vi "Qualify Library Icon Core.vi"(0 "VI Reference":refnum<vi>, 11 "error in":errorcluster) -> (3 "Class?":bool, 4 "Good Library Icon":bool, 6 "Maximum Number of Rows":i32, 8 "Library Path":path, 10 "Number of Rows in Icon":i32, 14 "Icon Image":picture, 15 "error out":errorcluster)   [LabVIEW 2020, in "Text-Based VI Icon.lvlib"]
uses:
  Text-Based VI Icon.lvlib
panel:
  out "Left and Right Good (for Debugging)":bool
  out "Top and Bottom Good (for Debugging)":bool
  out "Good Frame Color (for Debugging)":bool
  out "Supported Size or Shape (for Debugging)":bool
  out "Last True Mask + 1 (for Debugging)":i32
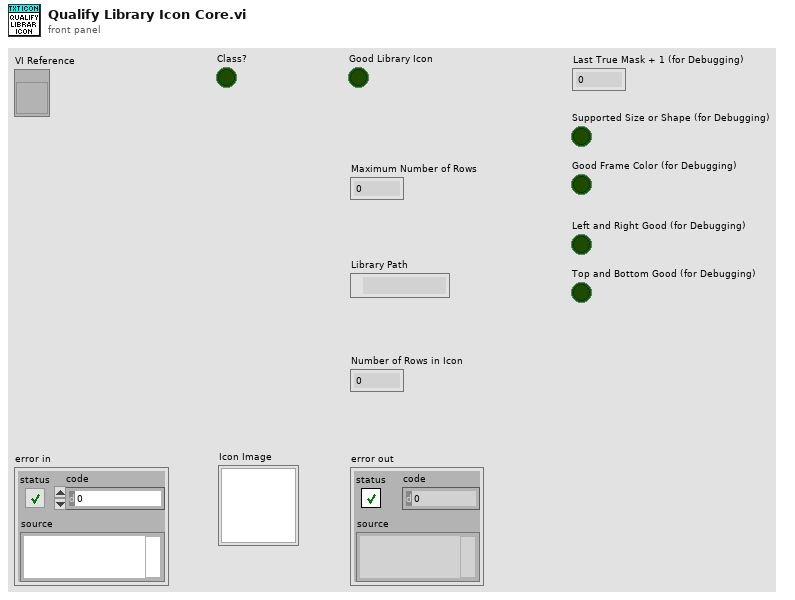
[diagram p1: front panel]
types:
  T1 = typedef "imagedata.ctl" = cluster{"image type":i32, "image depth":i32, "image":u8[], "mask":u8[], "colors":u32[], "Rectangle":cluster{"left":i16, "top":i16, "right":i16, "bottom":i16}}
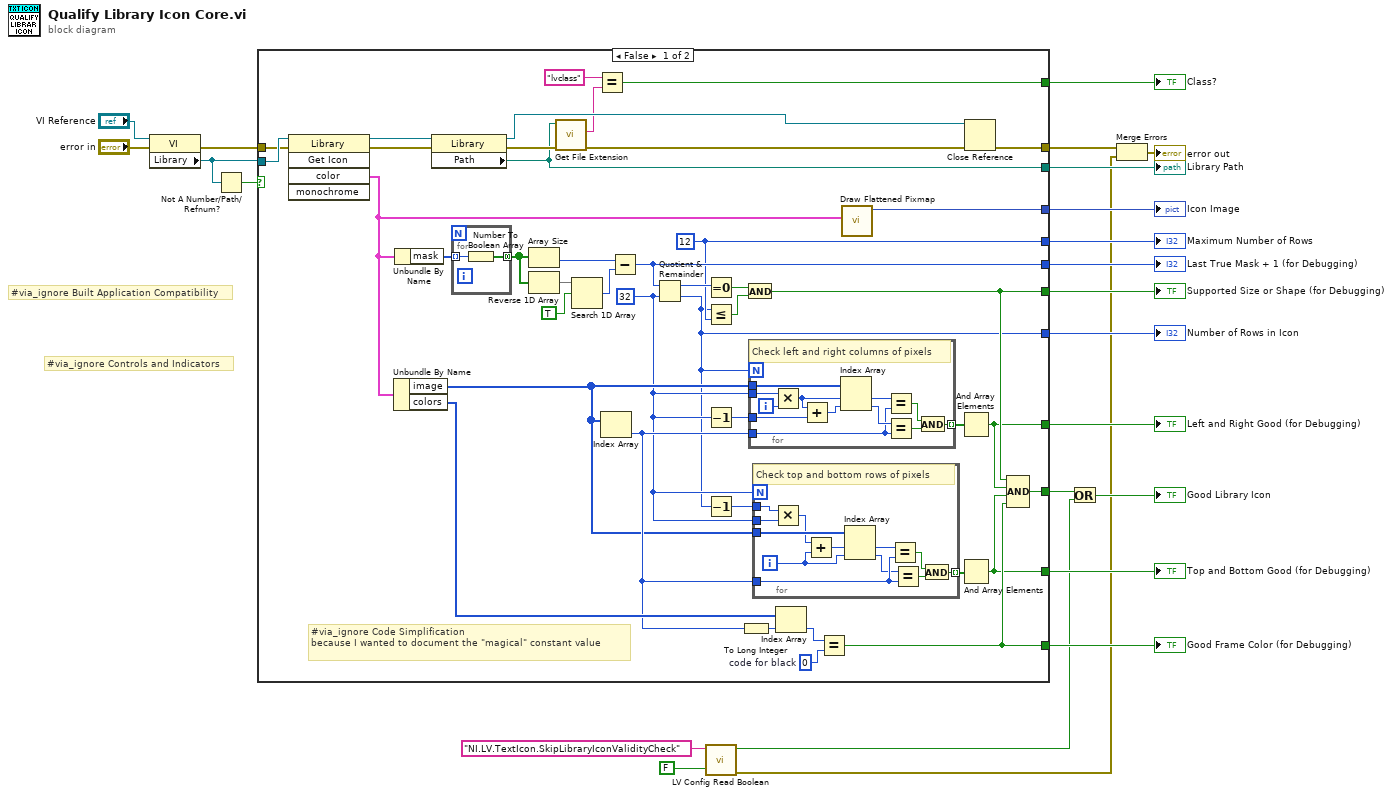
[diagram p0: block diagram]
diagram:
  # "#via_ignore Built Application Compatibility"
  # "#via_ignore Controls and Indicators"
  n1 = property class="VI"(reference="VI Reference", error in="error in") -> (error out=w21:errorcluster, "Library"=w22:refnum<vi>)  [unwired: 1 out]
  n2 = Not A Number/Path/Refnum?(number/path/refnum=w22) -> (NaN/Path/Refnum?=w23:bool)
  n3 = case shown="False" w23 {
    tunnel: w22 -> [w65 _]
    tunnel: w21 -> [w64 w92]
    tunnel: [w33 w92] -> w3
    tunnel: [w54 _] -> w20
    tunnel: [w41 _] -> w19
    tunnel: [w39 _] -> w18
    tunnel: [w38 _] -> w17
    tunnel: [w40 _] -> w16
    tunnel: [w42 _] -> w15
    tunnel: [w37 _] -> w5
    tunnel: [w26 _] -> w14
    tunnel: [w34 _] -> w11
    tunnel: [w27 _] -> w10
    tunnel: [w24 _] -> w9
    frame False {
      w52 = u32 0  # code for black
      w34 = 12 ("y")
      w43 = 32 ("y")
      # "#via_ignore Code Simplification\nbecause I wanted to document the \"magical\" constant value"
      n4 = invoke class="Library" method="Get Icon"(reference=w65, error in=w64) -> (reference out=w36:refnum<vi>, error out=w35:errorcluster, "color"=w25:T1)  [unwired: 3 in, 2 out]
      n5 = Unbundle By Name(w25) -> ("image"=w47:u8[], "colors"=w53:u32[])
      n6 = Unbundle By Name(w25) -> ("mask"=w60:u8[])
      n7 = property class="Library"(reference=w36, error in=w35) -> (reference out=w32:refnum<vi>, error out=w31:errorcluster, "Path"=w26:path)
      n8 = for {
        tunnel: w60 -> [w91] mode=indexing
        tunnel: [w90] -> w57 mode=concatenating
        n9 = Number To Boolean Array(number=w91) -> (Boolean array=w90:bool[])
      }
      n10 = Array Size(array=w57) -> (size(s)=w56:i32)
      n11 = Reverse 1D Array(array=w57) -> (reversed array=w59:bool[])
      n12 = call <vilib>:"Get File Extension.vi"("error in (no error)"=w31, "file"=w26) -> ("error out"=w30:errorcluster, "lowercase file extension"=w29:string)  [unwired: 5 in, 3 out]
      n13 = Search 1D Array(1D array=w59, element=TRUE) -> (index of element=w55:i32)  [unwired: 1 in]
      n14 = Equal?(x="lvclass", y=w29) -> (x = y?=w27:bool)
      n15 = Index Array(array=w47) -> (element=w48:u8)  [unwired: 1 in]
      n16 = Subtract(x=w56, y=w55) -> (x-y=w54:i32)
      n17 = Quotient & Remainder(x=w54, y=w43) -> (x-y*floor(x/y)=w63:i32, floor(x/y)=w24:i32)
      n18 = Equal To 0?(x=w63) -> (x = 0?=w62:bool)
      n19 = Less Or Equal?(x=w24, y=w34) -> (x <= y?=w61:bool)
      n20 = Decrement(x=w43) -> (x-1=w45:i32)
      n21 = Decrement(x=w24) -> (x-1=w49:i32)
      n22 = To Long Integer(number=w48) -> (32bit integer=w51:i32)
      n23 = And(x=w62, y=w61) -> (x .and. y?=w41:bool)
      n24 = for {
        N: w24 -> [_]
        tunnel: w48 -> [w79]
        tunnel: [w87] -> w46 mode=indexing
        tunnel: w45 -> [w85]
        tunnel: w47 -> [w83]
        tunnel: w43 -> [w81]
        i -> [w86]
        # "Check left and right columns of pixels"
        n25 = Multiply(x=w81, y=w86) -> (x*y=w78:i32)
        n26 = Add(x=w78, y=w85) -> (x+y=w80:i32)
        n27 = Index Array(array=w83, index #1=w78, index #2=w80) -> (element #1=w82:u8, element #2=w84:u8)
        n28 = Equal?(x=w82, y=w79) -> (x = y?=w89:bool)
        n29 = Equal?(x=w84, y=w79) -> (x = y?=w88:bool)
        n30 = And(x=w89, y=w88) -> (x .and. y?=w87:bool)
      }
      n31 = for {
        N: w43 -> [_]
        tunnel: w47 -> [w77]
        tunnel: w49 -> [w76]
        tunnel: w48 -> [w71]
        tunnel: [w67] -> w50 mode=indexing
        tunnel: w43 -> [w66]
        i -> [w73]
        # "Check top and bottom rows of pixels"
        n32 = Multiply(x=w76, y=w66) -> (x*y=w75:i32)
        n33 = Add(x=w75, y=w73) -> (x+y=w74:i32)
        n34 = Index Array(array=w77, index #1=w74, index #2=w73) -> (element #1=w72:u8, element #2=w70:u8)
        n35 = Equal?(x=w72, y=w71) -> (x = y?=w69:bool)
        n36 = Equal?(x=w70, y=w71) -> (x = y?=w68:bool)
        n37 = And(x=w69, y=w68) -> (x .and. y?=w67:bool)
      }
      n38 = Index Array(array=w53, index=w51) -> (element=w44:u32)
      n39 = Equal?(x=w44, y=w52) -> (x = y?=w39:bool)
      n40 = call <vilib>:"Draw Flattened Pixmap.vi"("image data"=w25) -> ("new picture"=w42:picture)  [unwired: 8 in]
      n41 = And Array Elements(Boolean array=w46) -> (logical AND=w40:bool)
      n42 = And Array Elements(Boolean array=w50) -> (logical AND=w38:bool)
      n43 = Close Reference(reference=w32, error in (no error)=w30) -> (error out=w33:errorcluster)
      n44 = Compound Arithmetic op=AND(w41, w40, w38, w39) -> (w37:bool)
    }
    frame True {
    }
  }
  "Last True Mask + 1 (for Debugging)" <- w20
  "Supported Size or Shape (for Debugging)" <- w19
  "Good Frame Color (for Debugging)" <- w18
  "Top and Bottom Good (for Debugging)" <- w17
  "Left and Right Good (for Debugging)" <- w16
  "Icon Image" <- w15
  "Library Path" <- w14
  "Maximum Number of Rows" <- w11
  "Class?" <- w10
  "Number of Rows in Icon" <- w9
  n45 = call <resource>:"LV Config Read Boolean.vi"("default value"=FALSE, "key"="NI.LV.TextIcon.SkipLibraryIconValidityCheck") -> ("error out"=w2:errorcluster, "value"=w6:bool)  [unwired: 3 in, 1 out]
  n46 = Or(x=w5, y=w6) -> (x .or. y?=→"Good Library Icon":bool)
  n47 = Merge Errors(w3, w2) -> (→"error out":errorcluster)
